vi "origin_distance (SubVI).vi"(8 "error in (no error)":errorcluster, 10 "Origin Pixel":cluster{"X":sgl, "Y":sgl}, 11 "Refnum in":T1) -> (0 "error out":errorcluster, 1 "Number of Particles":i32, 2 "Array":string[](array[string]), 3 "Array of Real World Coordinates":cluster{"X":sgl, "Y":sgl}[](array[cluster]))   [LabVIEW 2020]
uses:
  <vilib>/vision/Image Controls.llb/IMAQ Image.ctl
  <vilib>/vision/NI_Vision_Development_Module.lvlib
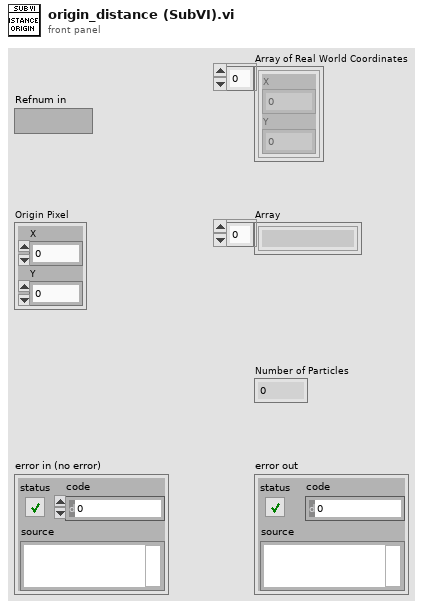
[diagram p1: front panel]
types:
  T1 = typedef "IMAQ Image.ctl" = refnum<image>
  T2 = cluster{"Area":dbl, "Number of Holes":dbl, "Bounding Rect":cluster{"Left":dbl, "Top":dbl, "Right":dbl, "Bottom":dbl}, "Center of Mass":cluster{"X":dbl, "Y":dbl}, "Orientation":dbl, "Dimensions":cluster{"Width":dbl, "Height":dbl}}[]
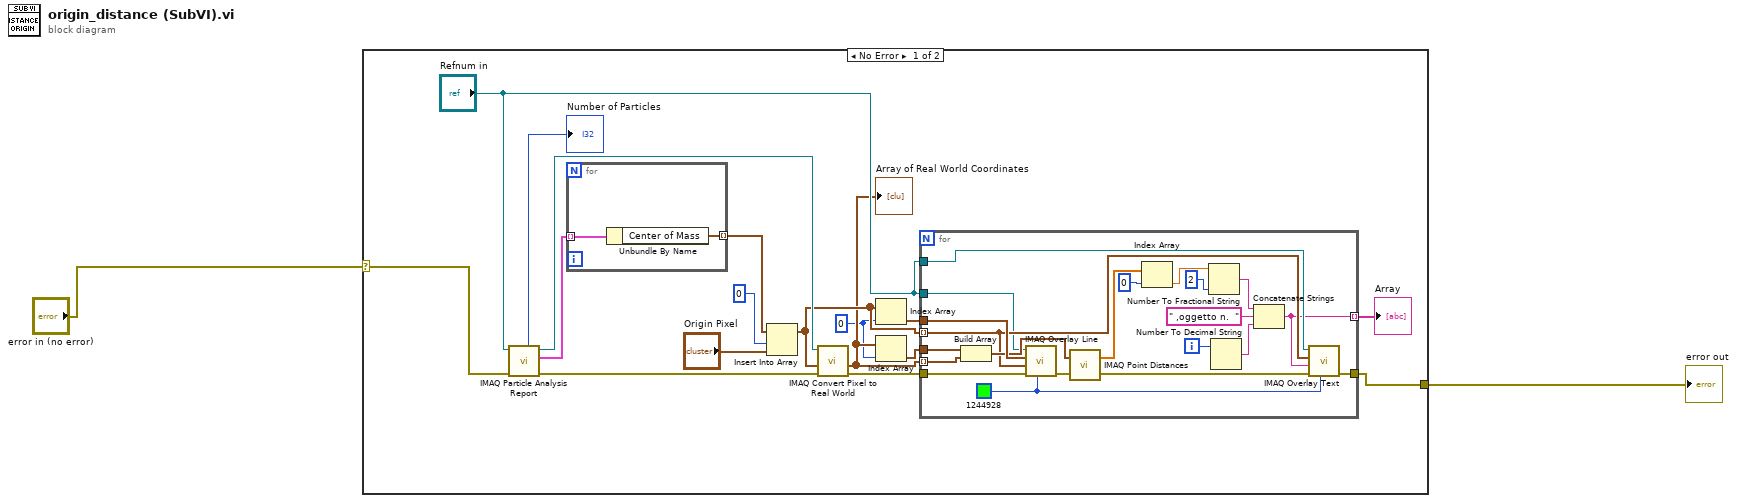
[diagram p0: block diagram]
diagram:
  n1 = case shown="No Error" "error in (no error)" {
    selector: "error in (no error)" -> [w4 w43]
    tunnel: [w3 w43] -> w1
    frame No Error {
      w7 = 0 ("index")
      n2 = call "IMAQ Particle Analysis Report"("error in (no error)"=w4, "Image"="Refnum in") -> ("error out"=w17:errorcluster, "Particle Reports (Pixels)"=w14:T2, "Image Out (duplicate)"=w15:T1, "Number of Particles"=→"Number of Particles":i32)  [unwired: 4 in, 2 out]
      n3 = for {
        tunnel: [w41] -> w10 mode=indexing
        tunnel: w14 -> [w42] mode=indexing
        n4 = Unbundle By Name(w42) -> ("Center of Mass"=w41:cluster{"X":dbl, "Y":dbl})
      }
      n5 = Insert Into Array(array=w10, index=0, new element="Origin Pixel") -> (w11:cluster{"X":dbl, "Y":dbl}[])
      n6 = call "IMAQ Convert Pixel to Real World"("error in (no error)"=w17, "Array of Pixel Coordinates"=w11, "Calibrated Image"=w15) -> ("error out"=w18:errorcluster, "Array of Real World Coordinates"=w9:cluster{"X":sgl, "Y":sgl}[])  [unwired: 3 in, 4 out]
      "Array of Real World Coordinates" <- w9
      n7 = Index Array(array=w11, index=w7) -> (element=w6:cluster{"X":dbl, "Y":dbl})
      n8 = Index Array(array=w9, index=w7) -> (element=w8:cluster{"X":sgl, "Y":sgl})
      n9 = for {
        tunnel: w11 -> [w34] mode=indexing
        tunnel: w6 -> [w40]
        tunnel: w8 -> [w37]
        tunnel: w9 -> [w35] mode=indexing
        tunnel: [w38] -> w3
        tunnel: "Refnum in" -> [w23]
        tunnel: "Refnum in" -> [w22]
        tunnel: w18 -> [w21]
        tunnel: [w20] -> w19 mode=indexing
        i -> [w29]
        w33 = u32 1244928 ("Color")
        n10 = Build Array(w37, w35) -> (w36:cluster{"X":sgl, "Y":sgl}[])
        n11 = call "IMAQ Overlay Line"("Color"=w33, "error in (no error)"=w21, "End Point"=w34, "Start Point"=w40, "Image"=w22) -> ("error out"=w39:errorcluster)  [unwired: 5 in, 1 out]
        n12 = call "IMAQ Point Distances"("Points"=w36, "error in (no error)"=w39) -> ("Distances"=w32:sgl[], "error out"=w25:errorcluster)  [unwired: 3 in]
        n13 = Index Array(array=w32, index=0) -> (element=w30:sgl)
        n14 = Number To Fractional String(number=w30, precision (6)=i16 2) -> (F-format string=w27:string)  [unwired: 2 in]
        n15 = Number To Decimal String(number=w29) -> (decimal integer string=w28:string)  [unwired: 1 in]
        n16 = Concatenate Strings(w27, " ,oggetto n.  " ("string"), w28) -> (w20:string)
        n17 = call "IMAQ Overlay Text"("Text Color (black)"=w33, "error in (no error)"=w25, "String"=w20, "Origin"=w34, "Image"=w23) -> ("error out"=w38:errorcluster)  [unwired: 5 in, 1 out]
      }
      "Array" <- w19
    }
    frame Error {
    }
  }
  "error out" <- w1
